vi "Get List Information.vi"(8 "List Selection":string, 9 "DQMH Modules Info":T2, 10 "References Map":map{string, refnum<vi>}(c390), 11 "Tree Map":T4) -> (0 "Documentation":T1, 1 "Module Type":T3, 2 "Vi out":refnum<vi>, 3 "Library name":string, 4 "VI Connector Pane":picture, 5 "DQMH Lib":refnum<vi>)   [LabVIEW 2020, in "Dashboard.lvlib"]
uses:
  Dashboard.lvlib
  <vilib>/National Instruments/Tree Map/Tree Map Data.ctl
  Module type--enum.ctl
  DQMH Modules Info--cluster.ctl
  Documentation--cluster.ctl
  <vilib>/National Instruments/Tree Map/Tree Map.lvlib
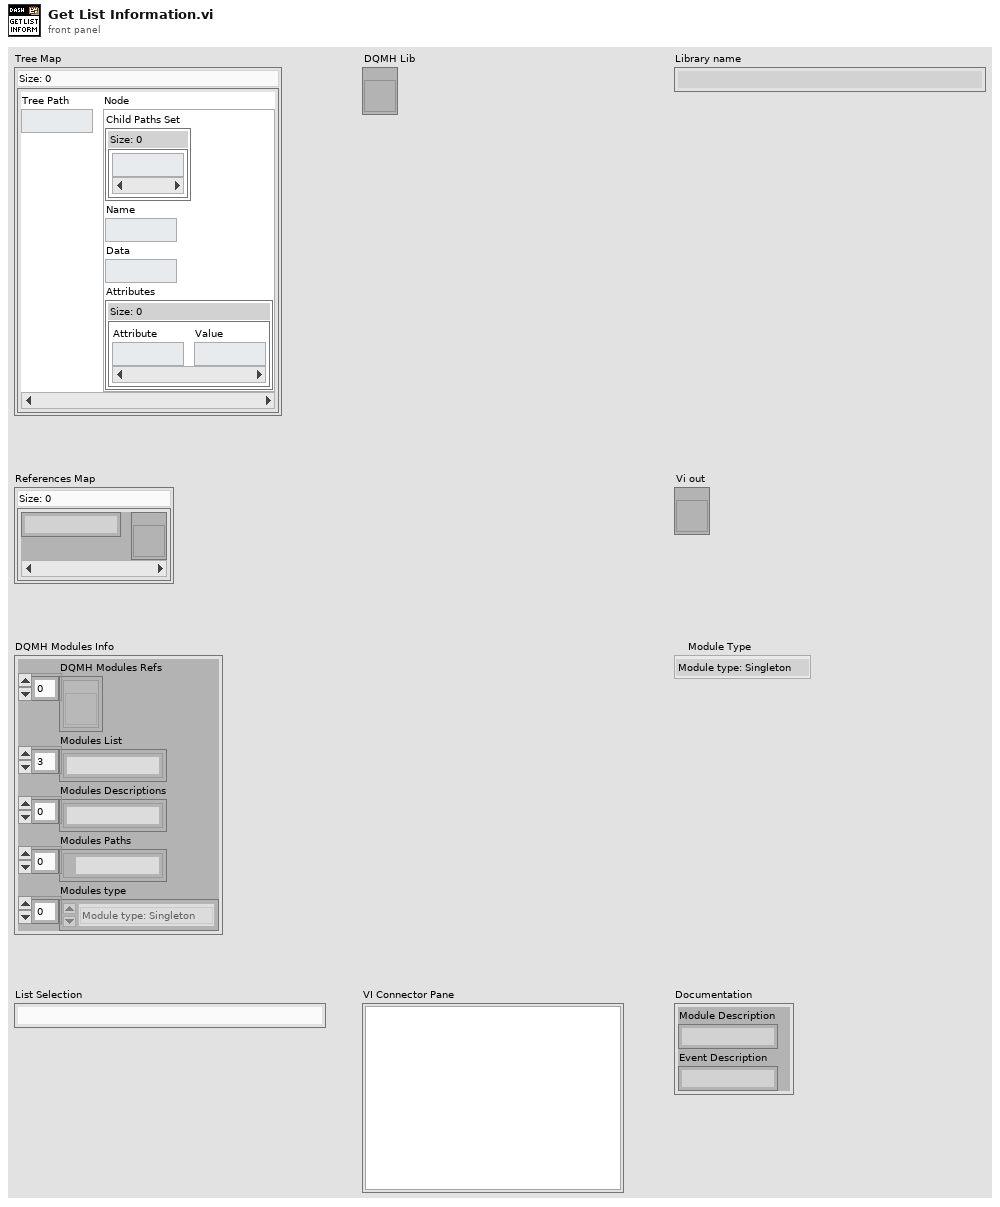
[diagram p1: front panel]
types:
  T1 = typedef "Dashboard.lvlib/Documentation--cluster.ctl" = cluster{"Module Description":string, "Event Description":string}
  T2 = typedef "Dashboard.lvlib/DQMH Modules Info--cluster.ctl" = cluster{"DQMH Modules Refs":refnum<vi>[], "Modules List":string[], "Modules Descriptions":string[], "Modules Paths":path[], "Modules type":T3[]}
  T3 = typedef "Dashboard.lvlib/Module type--enum.ctl" = enum16{"Module type: Singleton", "Module type: Cloneable"}
  T4 = typedef "Tree Map.lvlib/Tree Map Data.ctl" = map{string, cluster{"Child Paths Set":set{string}, "Name":string, "Data":string, "Attributes":map{string, string}}}
  T5 = cluster{"Child Paths Set":set{string}, "Name":string, "Data":string, "Attributes":map{string, string}}
  T6 = cluster{"Description":string, "VI Description":string}
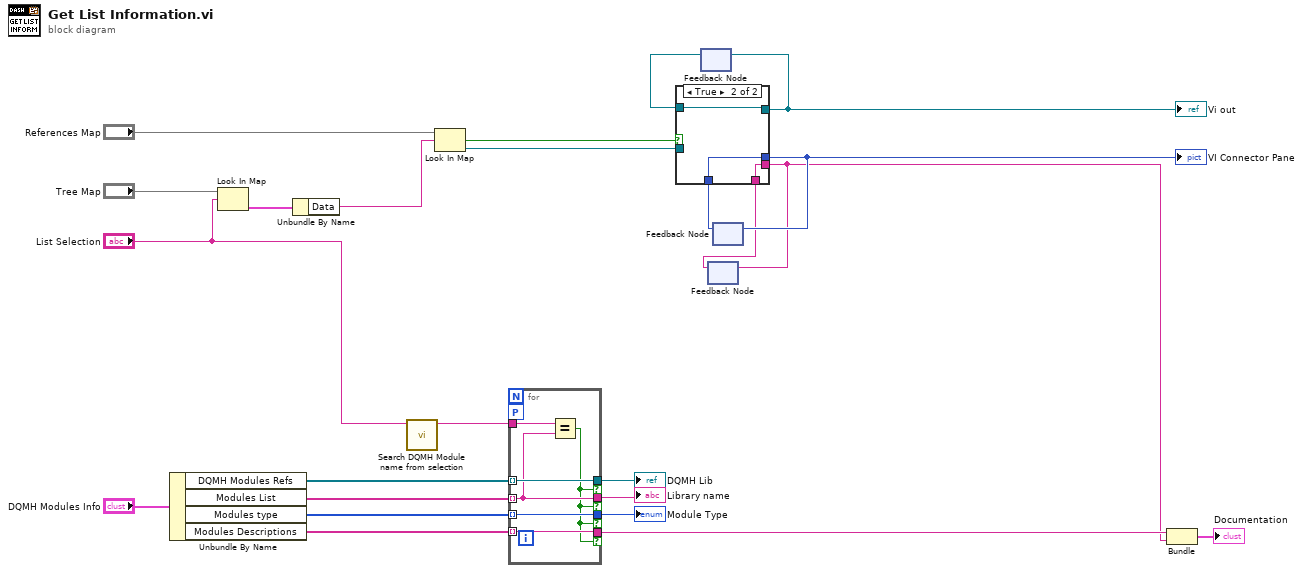
[diagram p0: block diagram]
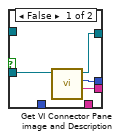
[diagram p2: hidden frame]
diagram:
  n1 = Unbundle By Name("DQMH Modules Info") -> ("DQMH Modules Refs"=w15:refnum<vi>[], "Modules List"=w16:string[], "Modules type"=w14:T3[], "Modules Descriptions"=w13:string[])
  n2 = Look In Map(map="Tree Map", key="List Selection") -> (value=w23:T5)  [unwired: 1 in, 1 out]
  n3 = Unbundle By Name(w23) -> ("Data"=w19:string)
  n4 = call "Search DQMH Module name from selection.vi"("Search Module Name"="List Selection") -> ("Module Name"=w12:string)  [unwired: 10 in]
  n5 = Look In Map(map="References Map", key=w19) -> (key not found?=w20:bool, value=w18:refnum<vi>)  [unwired: 1 in]
  n6 = for {
    tunnel: w16 -> [w28] mode=indexing
    tunnel: w15 -> [w29] mode=indexing
    tunnel: w14 -> [w27] mode=indexing
    tunnel: w13 -> [w26] mode=indexing
    tunnel: w12 -> [w30]
    tunnel: [w29] -> w7 if=w25
    tunnel: [w28] -> w11 if=w25
    tunnel: [w27] -> w10 if=w25
    tunnel: [w26] -> w9 if=w25
    workers-P: _ -> [_]
    n7 = Equal?(x=w30, y=w28) -> (x = y?=w25:bool)
  }
  "Module Type" <- w10
  "Library name" <- w11
  "DQMH Lib" <- w7
  n8 = feedback #1() -> (w5:refnum<vi>)  [unwired: 1 in]
  n9 = feedback #2() -> (w1:string)  [unwired: 1 in]
  n10 = feedback #3() -> (w3:picture)  [unwired: 1 in]
  n11 = case shown="True" w20 {
    tunnel: w18 -> [w34 _]
    tunnel: [w33 w36] -> w4
    tunnel: [w32 w37] -> w6
    tunnel: [w31 w35] -> w2
    tunnel: w5 -> [_ w37]
    tunnel: w3 -> [_ w36]
    tunnel: w1 -> [_ w35]
    frame False {
      n12 = call "Get VI Connector Pane image and Description.vi"("VI in"=w34) -> ("VI Description"=w31:string, "VI Connector Pane"=w33:picture, "Vi out"=w32:refnum<vi>)  [unwired: 7 in, 1 out]
    }
    frame True {
    }
  }
  "VI Connector Pane" <- w4
  "Vi out" <- w6
  n13 = feedback-in #1(w6) -> ()
  n14 = feedback-in #2(w2) -> ()
  n15 = feedback-in #3(w4) -> ()
  n16 = Bundle("Description"=w9, "VI Description"=w2) -> (→"Documentation":T6)  [unwired: 1 in]
